vi "IsSoftwareSetInstallable.vi"(8 "error in (no error)":errorcluster, 10 "Software Set ID":string, 11 "Session in":refnum<k21>) -> (0 "error out":errorcluster, 1 "Broken Dependencies":T1[](array[typedef]) {"dependee"."component type" items=["standard", "hidden", "system", "unknown", "startup", "image", "essential"]; "depender"."component type" items=["standard", "hidden", "system", "unknown", "startup", "image", "essential"]}, 2 "Is Installable":bool, 3 "Session out":refnum<k21>, 4 "Missing Add-ons":T1[](array[typedef]) {"dependee"."component type" items=["standard", "hidden", "system", "unknown", "startup", "image", "essential"]; "depender"."component type" items=["standard", "hidden", "system", "unknown", "startup", "image", "essential"]}, 5 "Deps Between Add-ons":T1[](array[typedef]) {"dependee"."component type" items=["standard", "hidden", "system", "unknown", "startup", "image", "essential"]; "depender"."component type" items=["standard", "hidden", "system", "unknown", "startup", "image", "essential"]}, 6 "installable addons":T4[](array[typedef]) {"Visibility Type" items=["standard", "hidden", "system", "unknown", "startup", "image", "essential"]})   [LabVIEW 2017, in "nisyscfg.lvlib"]
uses:
  <vilib>/nisyscfg/nisyscfg.lvlib
  <vilib>/nisyscfg/Broken Dependency 1.2.ctl
  <vilib>/nisyscfg/Software 1.2.ctl
  <vilib>/nisyscfg/Component Type.ctl
  <vilib>/nisyscfg/Software Extended.ctl
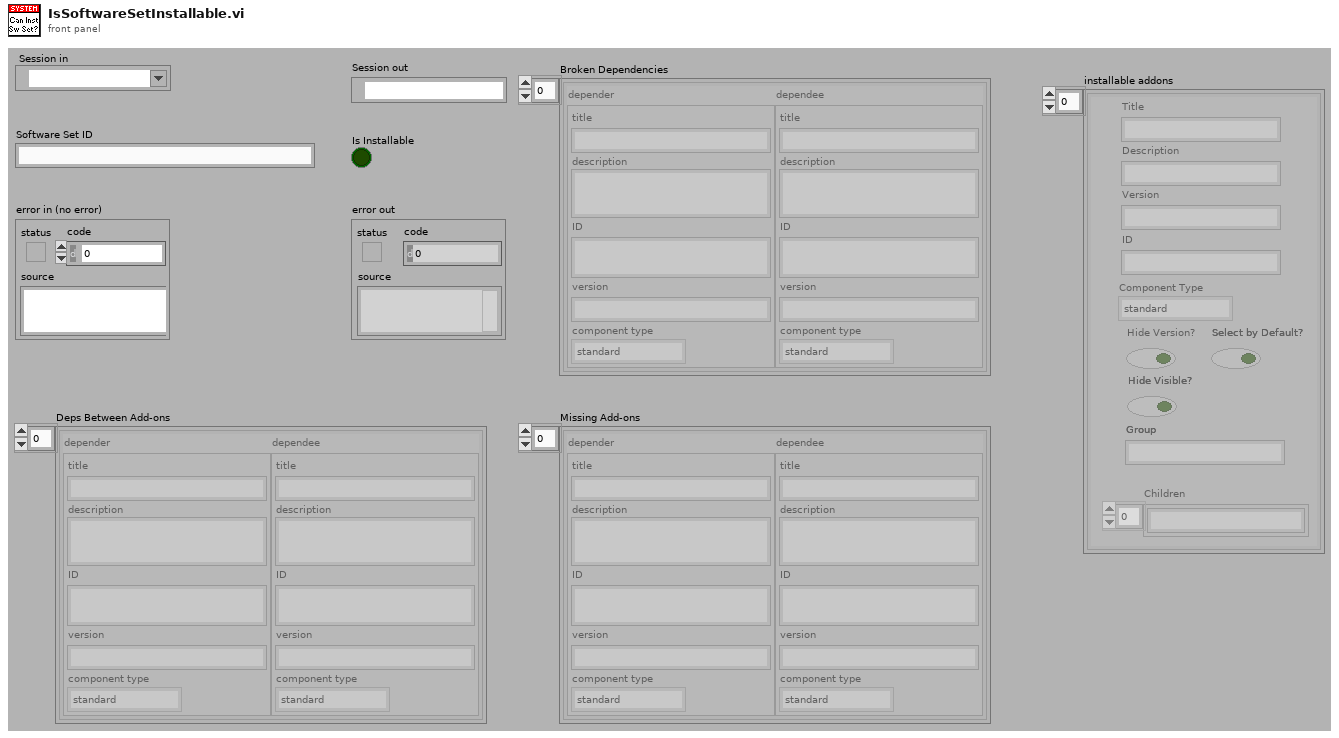
[diagram p1: front panel]
types:
  T1 = typedef "nisyscfg.lvlib/Broken Dependency 1.2.ctl" = cluster{"depender":T2, "dependee":T2}
  T2 = typedef "nisyscfg.lvlib/Software 1.2.ctl" = cluster{"title":string, "description":string, "ID":string, "version":string, "component type":T3}
  T3 = typedef "nisyscfg.lvlib/Component Type.ctl" = u32
  T4 = typedef "nisyscfg.lvlib/Software Extended.ctl" = cluster{"Description":string, "ID":string, "Version":string, "Title":string, "Visibility Type":T3, "Hide Version?":bool, "Children":string[], "Select by Default?":bool, "Hide Visible?":bool, "Group":string}
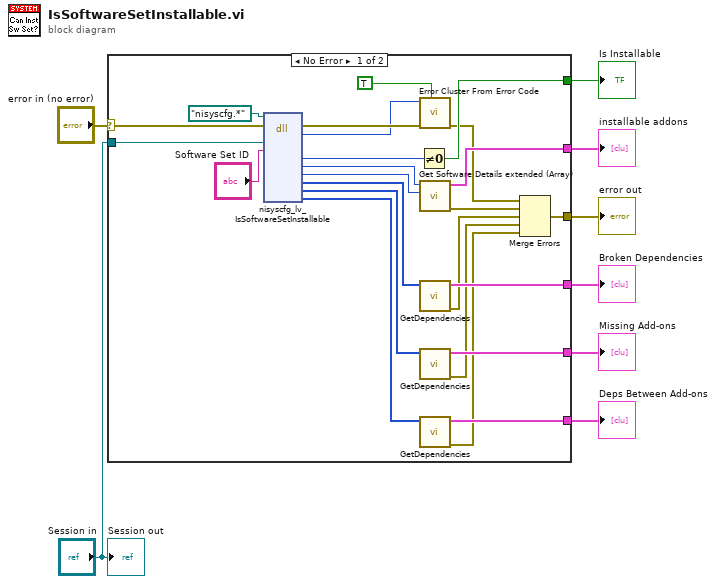
[diagram p0: block diagram]
diagram:
  n1 = case shown="No Error" "error in (no error)" {
    selector: "error in (no error)" -> [w27 w33]
    tunnel: "Session in" -> [w26 _]
    tunnel: [w28 _] -> w7
    tunnel: [w19 w33] -> w5
    tunnel: [w22 _] -> w4
    tunnel: [w15 _] -> w3
    tunnel: [w18 _] -> w2
    tunnel: [w17 _] -> w1
    frame No Error {
      n2 = dll-call lib="nisyscfg.*" fn="nisyscfg_lv_IsSoftwareSetInstallable" label="IsSoftwareSetInstallable"(path in=path "nisyscfg.*", error in=w27, "session"=w26, "softwareSetID"="Software Set ID") -> (error out=w31:errorcluster, "result"=w30:i32, "isInstallable"=w23:u8, "installableAddOns"=w16:u64, "numInstallableAddons"=w14:i32, "brokenDependencies"=w29:u64[], "missingAddOns"=w21:u64[], "depsBetweenAddOns"=w20:u64[])  [unwired: 9 in, 1 out]
      n3 = Not Equal To 0?(x=w23) -> (x != 0?=w22:bool)
      n4 = call <vilib>:"Error Cluster From Error Code.vi"("show call chain? (False)"=TRUE, "error in (no error)"=w31, "error code (0)"=w30) -> ("error out"=w13:errorcluster)  [unwired: 6 in]
      n5 = call <vilib>:"Get Software Details extended (Array).vi"("Number of Elements"=w14, "Enumerator in"=w16) -> ("error out"=w12:errorcluster, "Software Components"=w15:T4[])  [unwired: 8 in]
      n6 = call <vilib>:"GetDependencies.vi"("Enumerator in"=w29) -> ("error out"=w11:errorcluster, "Dependencies"=w28:T1[])  [unwired: 9 in]
      n7 = call <vilib>:"GetDependencies.vi"("Enumerator in"=w21) -> ("error out"=w10:errorcluster, "Dependencies"=w18:T1[])  [unwired: 9 in]
      n8 = call <vilib>:"GetDependencies.vi"("Enumerator in"=w20) -> ("error out"=w9:errorcluster, "Dependencies"=w17:T1[])  [unwired: 9 in]
      n9 = Merge Errors(w13, w12, w11, w10, w9) -> (w19:errorcluster)
    }
    frame Error {
    }
  }
  "error out" <- w5
  "Broken Dependencies" <- w7
  "Is Installable" <- w4
  "installable addons" <- w3
  "Missing Add-ons" <- w2
  "Deps Between Add-ons" <- w1
  "Session out" <- "Session in"
